vi "Get Control Captions.vi"(2 "error in":errorcluster, 3 "control refnums":refnum<vi>[](array[refnum])) -> (0 "error out":errorcluster, 1 "captions":string[](array[string]))   [LabVIEW 2020]
doc: "This VI controls the on/off state of 15 valves."
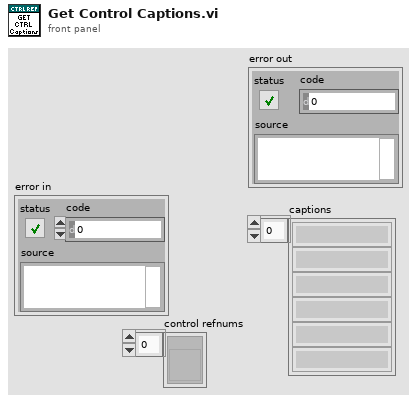
[diagram p1: front panel]
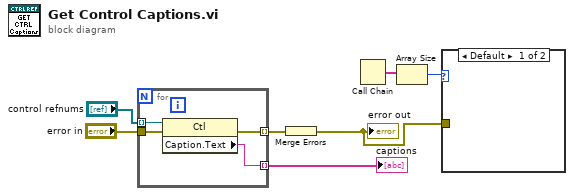
[diagram p0: block diagram]
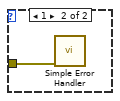
[diagram p2: hidden frame]
diagram:
  n1 = for {
    tunnel: [w8] -> w7 mode=indexing
    tunnel: "control refnums" -> [w10] mode=indexing
    tunnel: "error in" -> [w11]
    tunnel: [w9] -> w1 mode=indexing
    n2 = property on="Property Node" class="Ctl"(reference=w10, error in=w11) -> (error out=w9:errorcluster, "Caption.Text"=w8:string)  [unwired: 1 out]
  }
  "captions" <- w7
  n3 = Merge Errors(w1) -> (w4:errorcluster)
  "error out" <- w4
  n4 = Call Chain() -> (call chain=w2:string[])
  n5 = Array Size(array=w2) -> (size(s)=w3:i32)
  n6 = case shown="Default" w3 {
    tunnel: w4 -> [_ w12]
    frame Default {
    }
    frame 1 {
      n7 = call <vilib>:"Simple Error Handler.vi"("error in (no error)"=w12) -> ()  [unwired: 4 in, 5 out]
    }
  }
